vi "MRC IMU Get Yaw Landscape.vi"(8 "error in (no error)":errorcluster) -> (0 "error out":errorcluster, 1 "function return":i32, 2 "timestamp out":i64, 3 "yaw out":dbl)   [LabVIEW 2026, in "MrcLib.lvlib"]
doc: "MRC_Status MRC_CALLCONV MRC_IMU_GetYawLandscape(double* yaw, int64_t* timestamp);"
uses:
  <vilib>/MRC/MrcLib/MrcLib.lvlib
  MrcLib.dll
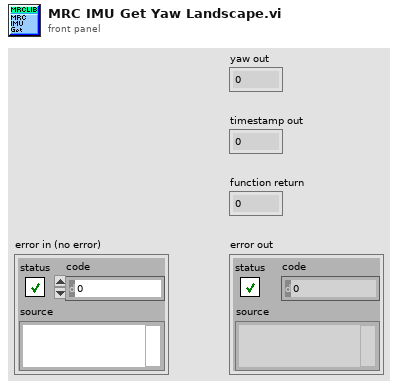
[diagram p1: front panel]
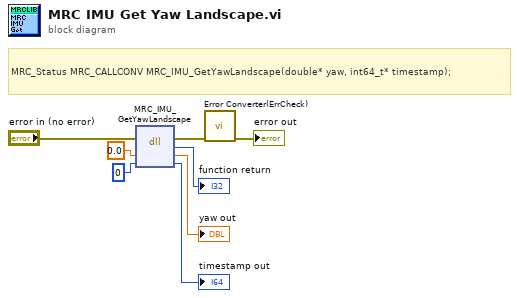
[diagram p0: block diagram]
diagram:
  # "MRC_Status MRC_CALLCONV MRC_IMU_GetYawLandscape(double* yaw, int64_t* timestamp);"
  n1 = dll-call lib="MrcLib.*" fn="MRC_IMU_GetYawLandscape"(error in="error in (no error)", "yaw"=0.0, "timestamp"=i64 0) -> (error out=w2:errorcluster, →"function return":i32, "yaw"=→"yaw out":dbl, "timestamp"=→"timestamp out":i64)  [unwired: 2 in, 1 out]
  n2 = call "Error Converter(ErrCheck).vi"("error in (no error)"=w2) -> ("error out"=→"error out":errorcluster)  [unwired: 10 in]
